vi "config crosslink test.vi"() -> (0 "error out":errorcluster, 2 "Editor crosslinked?":bool, 3 "Runtime crosslinked?":bool)   [LabVIEW 2014, in "Missing Plugin tests.lvlib"]
uses:
  Missing Plugin tests.lvlib
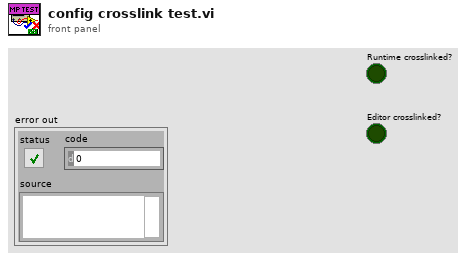
[diagram p1: front panel]
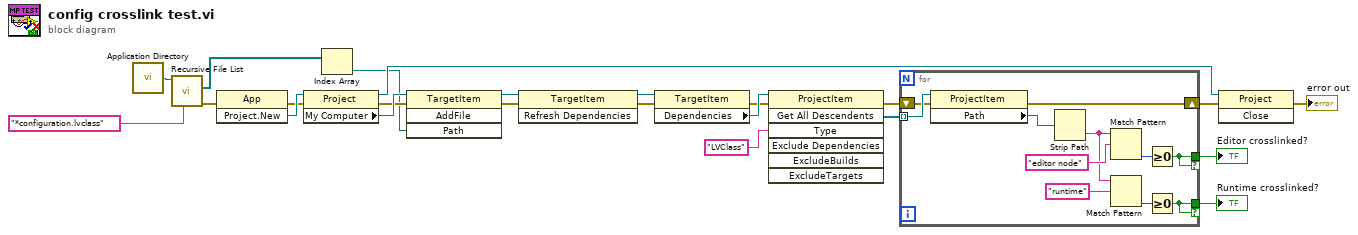
[diagram p0: block diagram]
diagram:
  n1 = call <vilib>:"Application Directory.vi"() -> ("Application Directory"=w6:path)
  n2 = call <vilib>:"Recursive File List.vi"("pattern"="*configuration.lvclass", "Folder Path"=w6) -> ("error out"=w2:errorcluster, "All Files in Dir"=w4:path[])  [unwired: 5 in, 3 out]
  n3 = invoke class="App" method="Project.New"(error in=w2) -> (error out=w17:errorcluster, "Project:New"=w20:refnum<vi>)  [unwired: 2 in, 1 out]
  n4 = property class="Project"(reference=w20, error in=w17) -> (reference out=w11:refnum<vi>, error out=w18:errorcluster, "My Computer"=w19:refnum<vi>)
  n5 = Index Array(array=w4) -> (element=w3:path)  [unwired: 1 in]
  n6 = invoke class="TargetItem" method="AddFile"(reference=w19, error in=w18, "Path"=w3) -> (reference out=w16:refnum<vi>, error out=w14:errorcluster)  [unwired: 1 in, 2 out]
  n7 = invoke class="TargetItem" method="Refresh Dependencies"(reference=w16, error in=w14) -> (reference out=w15:refnum<vi>, error out=w13:errorcluster)  [unwired: 1 in, 1 out]
  n8 = property class="TargetItem"(reference=w15, error in=w13) -> (error out=w9:errorcluster, "Dependencies"=w22:refnum<vi>)  [unwired: 1 out]
  n9 = invoke class="ProjectItem" method="Get All Descendents"(reference=w22, error in=w9, "Type"="LVClass") -> (error out=w10:errorcluster, "All Descendents"=w21:refnum<vi>[])  [unwired: 4 in, 5 out]
  n10 = for {
    tunnel: w21 -> [w34] mode=indexing
    shift-right: [w33] -> w12
    shift-left: w10 -> [w32]
    tunnel: [w25] -> w7 if=w25
    tunnel: [w24] -> w1 if=w24
    n11 = property class="ProjectItem"(reference=w34, error in=w32) -> (error out=w33:errorcluster, "Path"=w31:path)  [unwired: 1 out]
    n12 = Strip Path(path=w31) -> (name=w28:string)  [unwired: 1 out]
    n13 = Match Pattern(string=w28, regular expression="editor node") -> (offset past match=w29:i32)  [unwired: 1 in, 3 out]
    n14 = Match Pattern(string=w28, regular expression="runtime") -> (offset past match=w26:i32)  [unwired: 1 in, 3 out]
    n15 = Greater Or Equal To 0?(x=w29) -> (x >= 0?=w25:bool)
    n16 = Greater Or Equal To 0?(x=w26) -> (x >= 0?=w24:bool)
  }
  "Editor crosslinked?" <- w7
  "Runtime crosslinked?" <- w1
  n17 = invoke class="Project" method="Close"(reference=w11, error in=w12) -> (error out=→"error out":errorcluster)  [unwired: 1 in, 2 out]
